vi "See Elements Left.vi"(0 "object in":refnum<class "ExperimentSeries2.lvclass">, 5 "error in (no error)":errorcluster) -> (14 "object out":refnum<class "ExperimentSeries2.lvclass">, 16 "# elements in queue":i32, 17 "Elapsed Time":dbl format="%<%H:%M:%S>t", 18 "Time Left":dbl format="%<%H:%M:%S>t", 19 "error out":errorcluster)   [LabVIEW 2021, in "ExperimentSeries2.lvclass"]
uses:
  ExperimentSeries2.lvclass
  ExperimentSeries2.lvclass/ExperimentSeries2.ctl
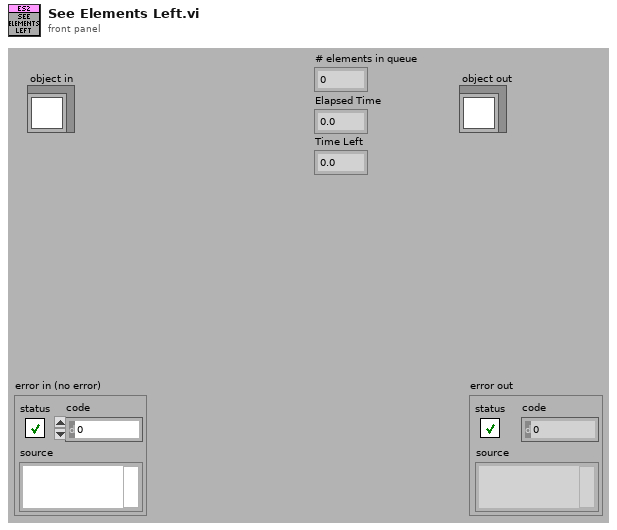
[diagram p1: front panel]
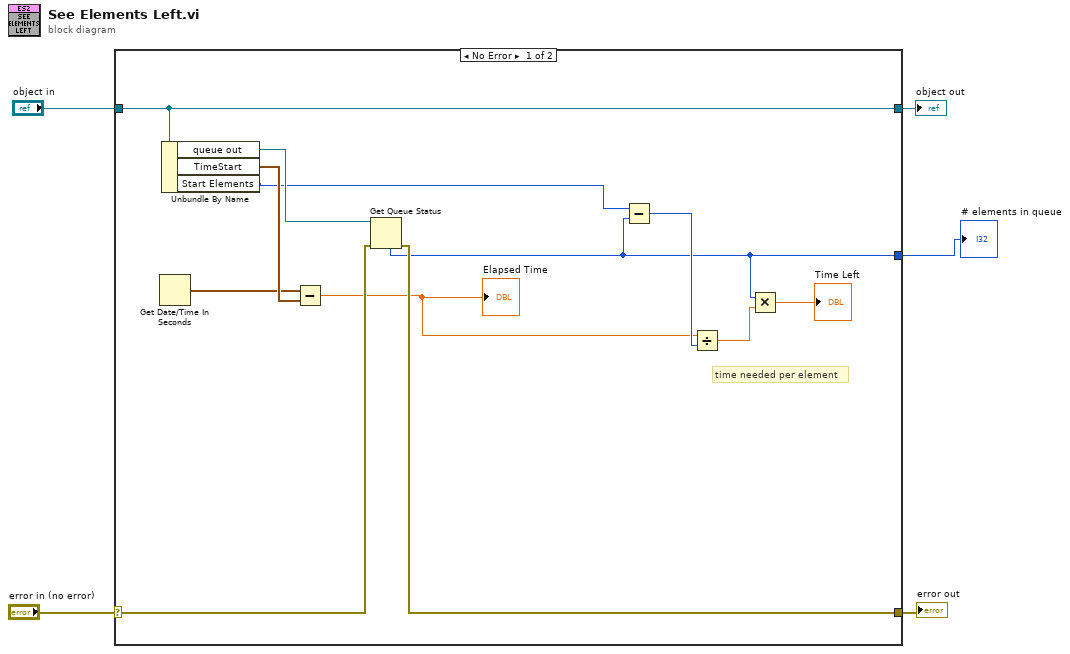
[diagram p0: block diagram]
diagram:
  n1 = case shown="No Error" "error in (no error)" {
    selector: "error in (no error)" -> [w16 w19]
    tunnel: [w15 w19] -> w4
    tunnel: [w17 w18] -> w2
    tunnel: "object in" -> [w17 w18]
    tunnel: [w8 _] -> w1
    frame No Error {
      # "time needed per element"
      n2 = Get Date/Time In Seconds() -> (seconds since 1Jan1904=w12:timestamp)
      n3 = Unbundle By Name(w17) -> ("queue out"=w14:refnum<queue>, "TimeStart"=w13:timestamp, "Start Elements"=w11:i32)
      n4 = Subtract(x=w12, y=w13) -> (x-y=w7:dbl)
      "Elapsed Time" <- w7
      n5 = Get Queue Status(queue=w14, error in (no error)=w16) -> (error out=w15:errorcluster, # elements in queue=w8:i32)  [unwired: 1 in, 6 out]
      n6 = Subtract(x=w11, y=w8) -> (x-y=w10:i32)
      n7 = Divide(x=w7, y=w10) -> (x/y=w9:dbl)
      n8 = Multiply(x=w8, y=w9) -> (x*y=→"Time Left":dbl)
    }
    frame Error {
    }
  }
  "error out" <- w4
  "object out" <- w2
  "# elements in queue" <- w1
